vi "AcquireImage test.vi"() -> ()   [LabVIEW 2009]
uses:
  Camera.lvlib
  ImageProcessing.lvlib
  ImageAnalysis.lvlib
  <vilib>/vision/NI_Vision_Development_Module.lvlib
panel:
  out "Major Radius":dbl
  out "Distance sideways":dbl
  out "Distance":dbl
  out "Ellipses":T1(array[cluster]) {"Position"."Y" format="%.2f"; "Position"."X" format="%.2f"}
  out "Image":T2(plugin-control)
  out "Objects bottom cords":cluster{"Cord":cluster{"X":dbl, "Y":dbl}[]}[](array[cluster])
  in  "stop":bool
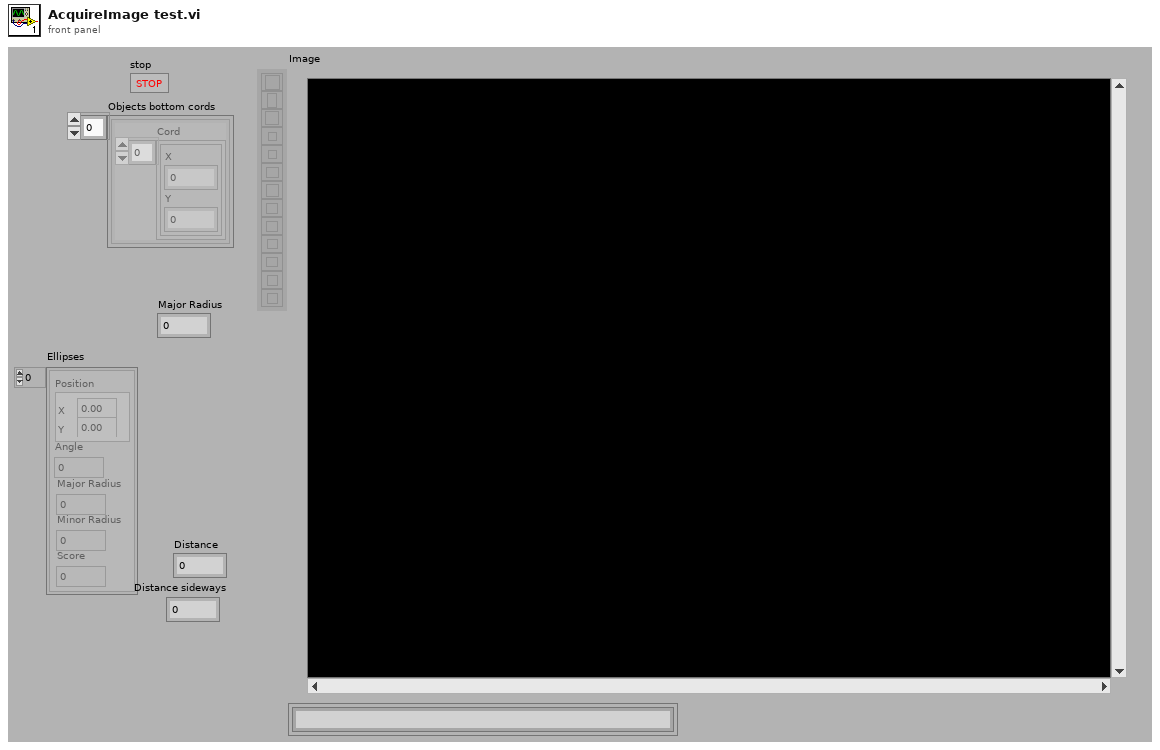
[diagram p1: front panel]
types:
  T1 = cluster{"Position":cluster{"X":sgl, "Y":sgl}, "Angle":dbl, "Major Radius":dbl, "Minor Radius":dbl, "Score":dbl}[]
  T2 = typedef "IMAQ Image.ctl" = refnum<image>
  T3 = cluster{"Position":cluster{"X":sgl, "Y":sgl}, "Angle":dbl, "Major Radius":dbl, "Minor Radius":dbl, "Score":dbl}
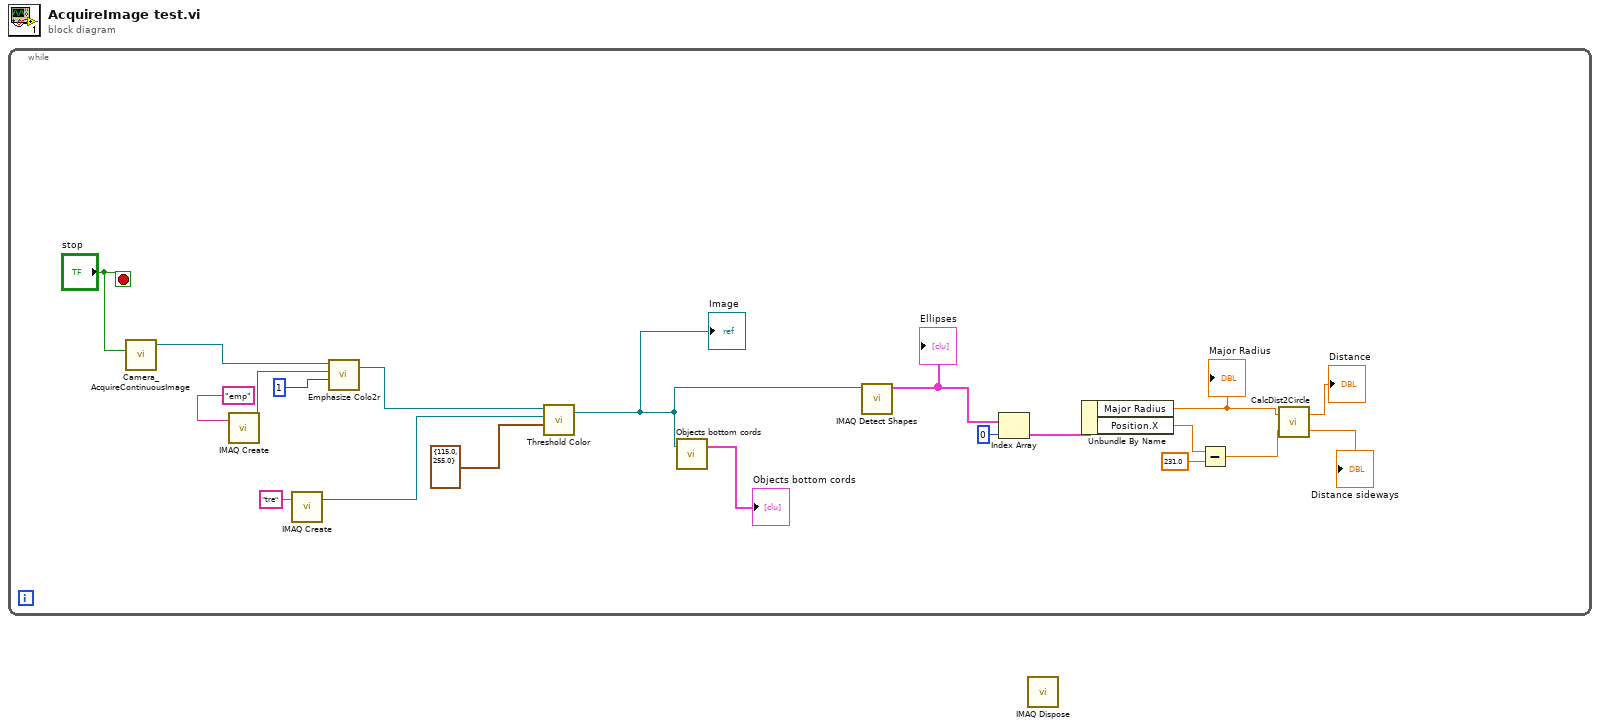
[diagram p0: block diagram]
diagram:
  n1 = while {
    stop <- "stop" stop-if-true
    n2 = call "Camera_AcquireContinuousImage.vi"("Stop (F)"="stop") -> ("Image Out"=w16:T2)  [unwired: 1 in, 2 out]
    n3 = call "IMAQ Create"("Image Name"="emp") -> ("New Image"=w18:T2)  [unwired: 4 in, 1 out]
    n4 = call "IMAQ Create"("Image Name"="tre") -> ("New Image"=w13:T2)  [unwired: 4 in, 1 out]
    n5 = call "Emphasize Colo2r.vi"("Color"=i8 1, "Image Dst"=w18, "Image Src"=w16) -> ("Image Out"=w12:T2)  [unwired: 1 in, 1 out]
    n6 = call "Threshold Color.vi"("Range"=cluster{"Lower value":sgl, "Upper value":sgl} {"Lower value"=115.0, "Upper value"=255.0}, "Image Dst"=w13, "Image Src"=w12) -> ("Image Dst Out"=w1:T2)  [unwired: 1 in, 1 out]
    "Image" <- w1
    n7 = call "Objects bottom cords.vi"("Image"=w1) -> ("Objects bottom cords"=→"Objects bottom cords":cluster{"Cord":cluster{"X":dbl, "Y":dbl}[]}[])  [unwired: 1 in, 1 out]
    n8 = call-poly "IMAQ Detect Shapes"("Image"=w1) -> ("Ellipses"=w3:T1)  [unwired: 8 in, 2 out]
    "Ellipses" <- w3
    n9 = Index Array(array=w3, index=0) -> (element=w2:T3)
    n10 = Unbundle By Name(w2) -> ("Major Radius"=w10:dbl, "Position.X"=w9:sgl)
    "Major Radius" <- w10
    n11 = Subtract(x=w9, y=sgl 231.0) -> (x-y=w7:sgl)
    n12 = call "CalcDist2Circle.vi"("Horizontal pixels from center"=w7, "Height of circle"=w10) -> ("Distance sideways"=→"Distance sideways":dbl, "Distance"=→"Distance":dbl)
  }
  n13 = call "IMAQ Dispose"() -> ()  [unwired: 6 in, 1 out]
